vi "Thorlabs_CCS_DisConnect.vi"(0 "VISA Refnum in":refnum<visa-resource-name>, 11 "error in (no error)":errorcluster) -> (15 "error out":errorcluster)   [LabVIEW 2021]
doc: "Disconnects the instrument by closing the VISA connection."
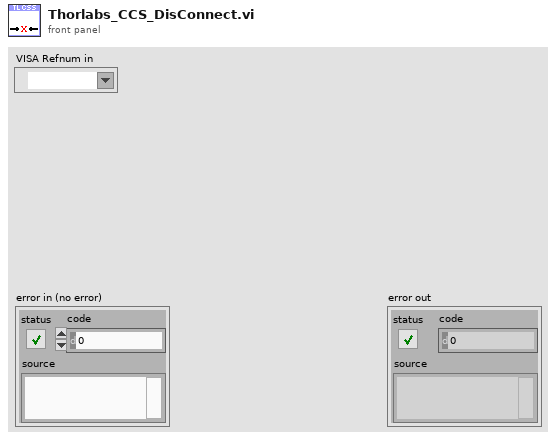
[diagram p1: front panel]
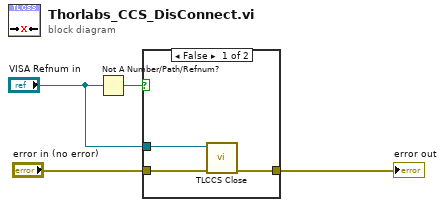
[diagram p0: block diagram]
diagram:
  n1 = Not A Number/Path/Refnum?(number/path/refnum="VISA Refnum in") -> (NaN/Path/Refnum?=w1:bool)
  n2 = case shown="False" w1 {
    tunnel: [w7 w8] -> w4
    tunnel: "VISA Refnum in" -> [w6 _]
    tunnel: "error in (no error)" -> [w5 w8]
    frame False {
      n3 = call <instrlib>:"TLCCS Close.vi"("error in (no error)"=w5, "instrument handle"=w6) -> ("error out"=w7:errorcluster)  [unwired: 9 in]
    }
    frame True {
    }
  }
  "error out" <- w4
